vi "QUERY_TELEM_ALL.vi"() -> ()   [LabVIEW 2023, in "Clover_Cell.lvlib"]
uses:
  Clover_Cell.lvlib
panel:
  out "AiP_8":dbl format="%#6.2f"
  out "AiP_7":dbl format="%#6.2f"
  out "AiP_6":dbl format="%#6.2f"
  out "AiP_5":dbl format="%#6.2f"
  out "AiP_4":dbl format="%#6.2f"
  out "AiP_3":dbl format="%#6.2f"
  out "AiP_2":dbl format="%#6.2f"
  out "AiP_1":dbl format="%#2.2f"
  out "Channel_56":i32
  out "Channel_55":i32
  out "Channel_54":i32
  out "Channel_53":i32
  out "Channel_52":i32
  out "Channel_51":i32
  out "Channel_50":i32
  out "Channel_49":i32
  out "Channel_40":i32
  out "Channel_39":i32
  out "Channel_38":i32
  out "Channel_37":i32
  out "Channel_36":i32
  out "Channel_35":i32
  out "Channel_34":i32
  out "Channel_33":i32
  out "Channel_24":i32
  out "Channel_23":i32
  out "Channel_22":i32
  out "Channel_21":i32
  out "Channel_20":i32
  out "Channel_19":i32
  out "Channel_18":i32
  out "Channel_17":i32
  out "Channel_8":i32
  out "Channel_7":i32
  out "Channel_6":i32
  out "Channel_5":i32
  out "Channel_4":i32
  out "Channel_3":i32
  out "Channel_2":i32
  out "Channel_1":i32
  out "L2_Pdet_Array":T1(array[cluster])
  in  "TRXmode":u16(ring)=1 items=["QUERY_TELEM_2 (V)"=2, "QUERY_TELEM_1 (H)"=1]
  in  "TCPIPin":T2={"address"="192.168.100.111", "remote port or service name"=5025, "timeout ms (60000)"=10000}
  out "size(s)":i32
  # "CLC_Gen4_L2"
  # "AiP_1 : 0\nAiP_2 : 1\nAiP_3 : 2\nAiP_4 : 3\nAiP_5 : 4\nAiP_6 : 5\nAiP_7 : 6\nAiP_8 : 7"
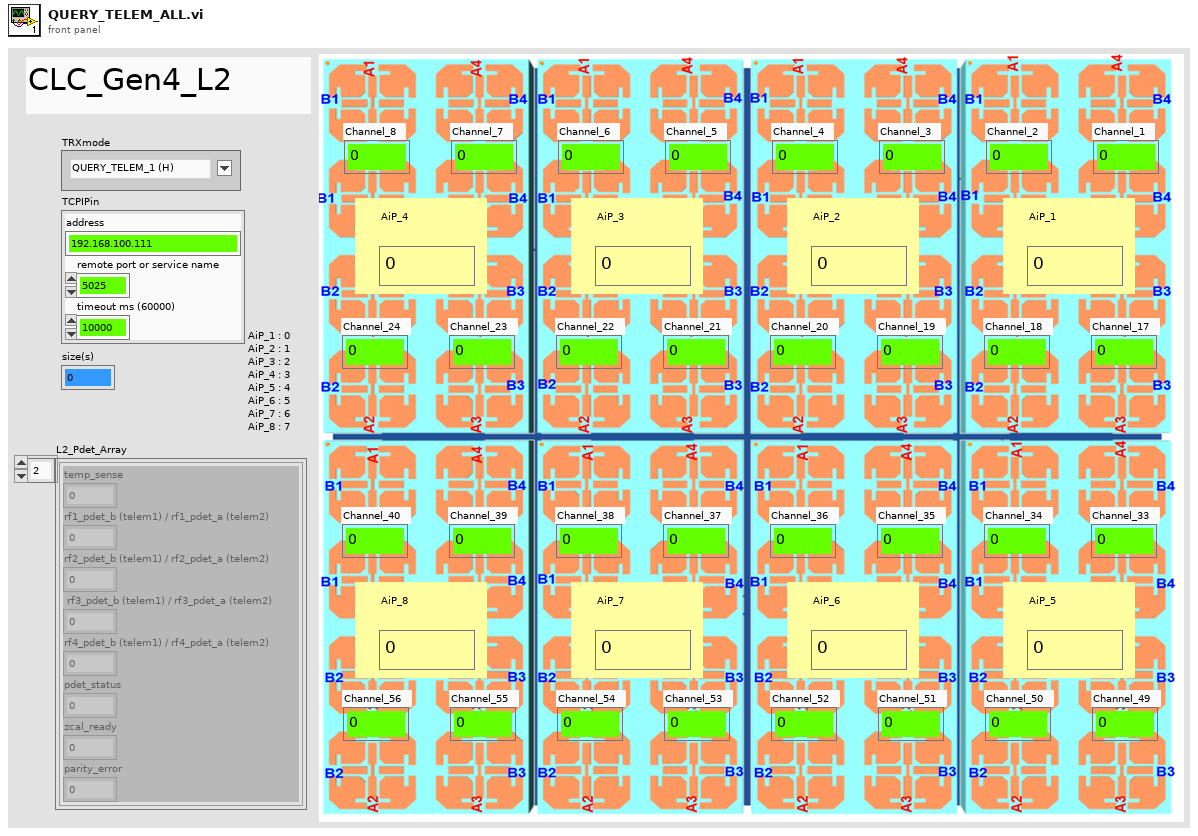
[diagram p1: front panel]
types:
  T1 = cluster{"temp_sense":i32, "rf1_pdet_b (telem1) / rf1_pdet_a (telem2)":i32, "rf2_pdet_b (telem1) / rf2_pdet_a (telem2)":i32, " rf3_pdet_b (telem1) / rf3_pdet_a (telem2)":i32, "rf4_pdet_b (telem1) / rf4_pdet_a (telem2)":i32, "pdet_status":i32, "zcal_ready":i32, "parity_error":i32}[]
  T2 = cluster{"address":string, "remote port or service name":u16, "timeout ms (60000)":i32}
  T3 = cluster{"temp_sense":i32, "rf1_pdet_b (telem1) / rf1_pdet_a (telem2)":i32, "rf2_pdet_b (telem1) / rf2_pdet_a (telem2)":i32, " rf3_pdet_b (telem1) / rf3_pdet_a (telem2)":i32, "rf4_pdet_b (telem1) / rf4_pdet_a (telem2)":i32, "pdet_status":i32, "zcal_ready":i32, "parity_error":i32}
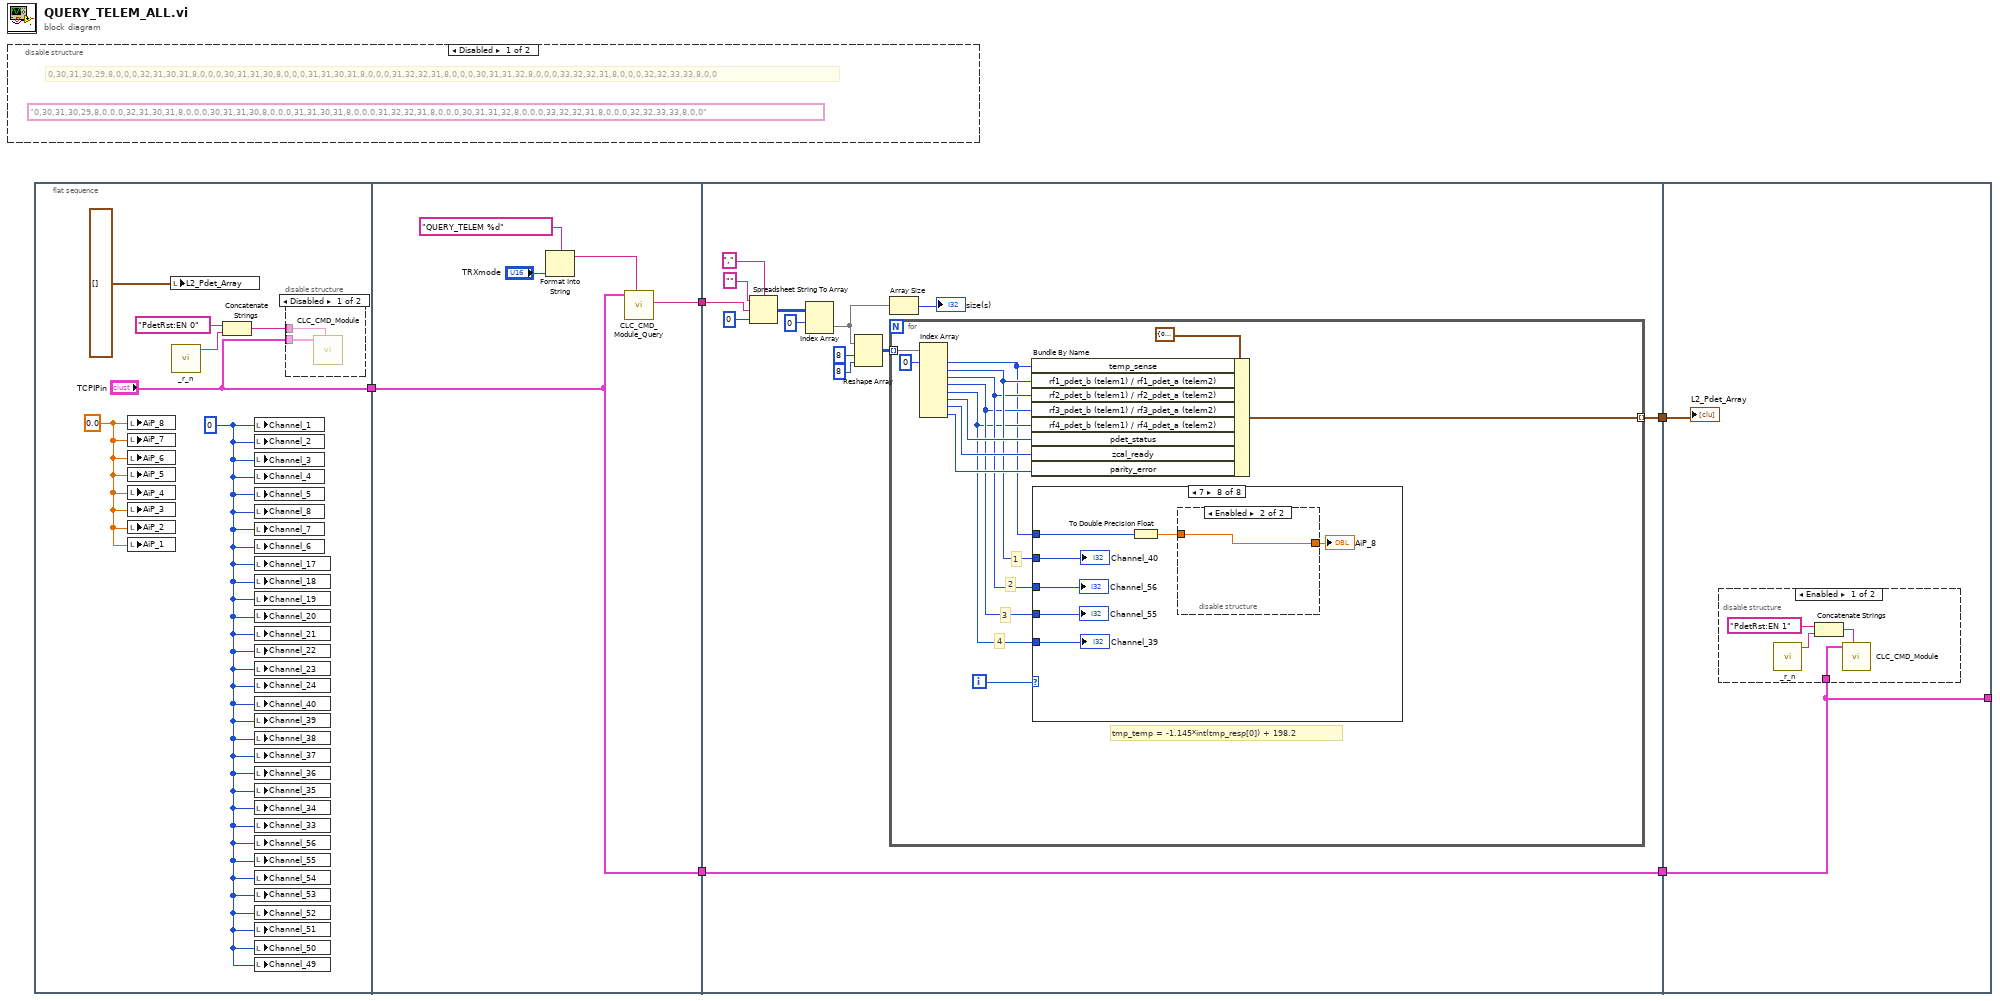
[diagram p0: block diagram]
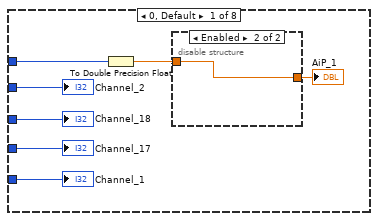
[diagram p4: hidden frame]
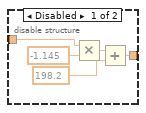
[diagram p5: hidden frame]
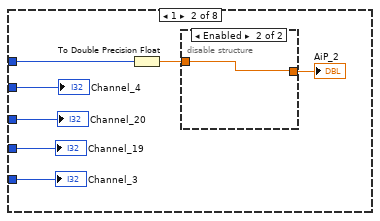
[diagram p6: hidden frame]
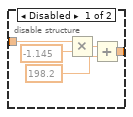
[diagram p7: hidden frame]
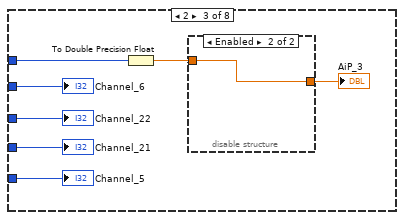
[diagram p8: hidden frame]
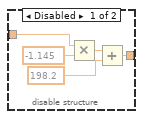
[diagram p9: hidden frame]
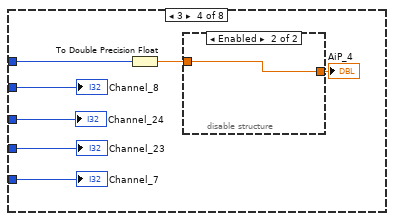
[diagram p10: hidden frame]
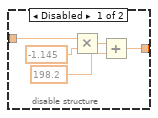
[diagram p11: hidden frame]
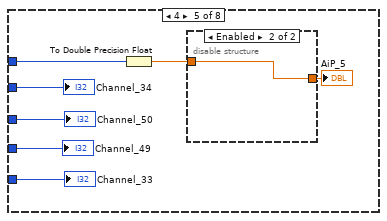
[diagram p12: hidden frame]
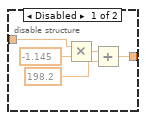
[diagram p13: hidden frame]
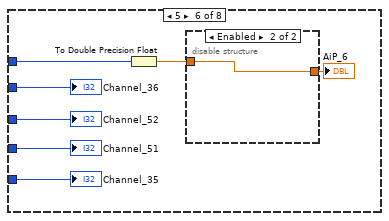
[diagram p14: hidden frame]
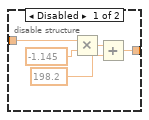
[diagram p15: hidden frame]
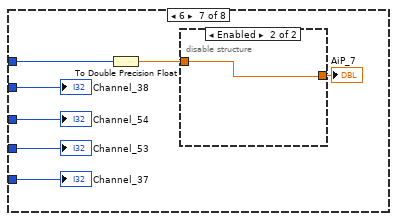
[diagram p16: hidden frame]
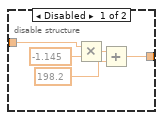
[diagram p17: hidden frame]
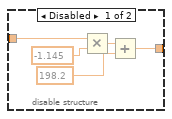
[diagram p18: hidden frame]
diagram:
  n1 = disable-structure shown="Disabled" {
    frame Disabled {
      (unwired) "0,30,31,30,29,8,0,0,0,32,31,30,31,8,0,0,0,30,31,31,30,8,0,0,0,31,31,30,31,8,0,0,0,31,32,32,31,8,0,0,0,30,31,31,32,8,0,0,0,33,32,32,31,8,0,0,0,32,32,33,33,8,0,0"
      # "0,30,31,30,29,8,0,0,0,32,31,30,31,8,0,0,0,30,31,31,30,8,0,0,0,31,31,30,31,8,0,0,0,31,32,32,31,8,0,0,0,30,31,31,32,8,0,0,0,33,32,32,31,8,0,0,0,32,32,33,33,8,0,0"
    }
    frame Enabled {
    }
  }
  n2 = flat-sequence {
    tunnel: ["TCPIPin"] -> w3
    tunnel: [w19] -> w5
    tunnel: [w15] -> w4
    tunnel: w3 -> [w15]
    tunnel: w5 -> [w30]
    tunnel: w4 -> [w21]
    tunnel: [w21] -> w2
    tunnel: [w20] -> w1
    tunnel: [w151] -> _
    tunnel: w2 -> [w151]
    tunnel: w1 -> [w150]
    frame #0 {
      w6 = 0.0 ("AiP_8")
      w7 = 0 ("Channel_1")
      n3 = local write "AiP_8"(w6) -> ()
      n4 = local write "AiP_7"(w6) -> ()
      n5 = local write "AiP_6"(w6) -> ()
      n6 = local write "AiP_5"(w6) -> ()
      n7 = local write "AiP_4"(w6) -> ()
      n8 = local write "AiP_3"(w6) -> ()
      n9 = local write "AiP_2"(w6) -> ()
      n10 = local write "AiP_1"(w6) -> ()
      n11 = local write "L2_Pdet_Array"(T1 [] ("L2")) -> ()
      n12 = call "_r_n.vi"() -> ("command"=w11:string)  [unwired: 5 in]
      n13 = Concatenate Strings("PdetRst:EN 0" ("CMD in"), w11) -> (w10:string)
      n14 = local write "Channel_1"(w7) -> ()
      n15 = local write "Channel_2"(w7) -> ()
      n16 = local write "Channel_3"(w7) -> ()
      n17 = local write "Channel_4"(w7) -> ()
      n18 = local write "Channel_5"(w7) -> ()
      n19 = local write "Channel_8"(w7) -> ()
      n20 = local write "Channel_7"(w7) -> ()
      n21 = local write "Channel_6"(w7) -> ()
      n22 = local write "Channel_17"(w7) -> ()
      n23 = local write "Channel_18"(w7) -> ()
      n24 = local write "Channel_19"(w7) -> ()
      n25 = local write "Channel_20"(w7) -> ()
      n26 = local write "Channel_21"(w7) -> ()
      n27 = local write "Channel_22"(w7) -> ()
      n28 = local write "Channel_23"(w7) -> ()
      n29 = local write "Channel_24"(w7) -> ()
      n30 = local write "Channel_40"(w7) -> ()
      n31 = local write "Channel_39"(w7) -> ()
      n32 = local write "Channel_38"(w7) -> ()
      n33 = local write "Channel_37"(w7) -> ()
      n34 = local write "Channel_36"(w7) -> ()
      n35 = local write "Channel_35"(w7) -> ()
      n36 = local write "Channel_34"(w7) -> ()
      n37 = local write "Channel_33"(w7) -> ()
      n38 = local write "Channel_56"(w7) -> ()
      n39 = local write "Channel_55"(w7) -> ()
      n40 = local write "Channel_54"(w7) -> ()
      n41 = local write "Channel_53"(w7) -> ()
      n42 = local write "Channel_52"(w7) -> ()
      n43 = local write "Channel_51"(w7) -> ()
      n44 = local write "Channel_50"(w7) -> ()
      n45 = local write "Channel_49"(w7) -> ()
      n46 = disable-structure shown="Disabled" {
        disable-tunnel: w10 -> [w14 _]
        disable-tunnel: "TCPIPin" -> [w13 _]
        frame Disabled {
          n47 = call "CLC_CMD_Module.vi"("CMD in"=w14, "TCPIPin"=w13) -> ()  [unwired: 6 in, 4 out]
        }
        frame Enabled {
        }
      }
    }
    frame #1 {
      n48 = Format Into String(format string="QUERY_TELEM %d" ("data in"), "TRXmode") -> (resulting string=w16:string)  [unwired: 2 in, 1 out]
      n49 = call "CLC_CMD_Module_Query.vi"("CMD in"=w16, "TCPIPin"=w15) -> ("data out"=w19:string)  [unwired: 7 in, 2 out]
    }
    frame #2 {
      n50 = Spreadsheet String To Array(delimiter (Tab)=",", format string="", spreadsheet string=w30, array type (2D Dbl)=0) -> (array=w26:i32[][])
      n51 = Index Array(array=w26, index (row)=0 ("disabled index (col)")) -> (element=w24:i32[])  [unwired: 1 in]
      n52 = Reshape Array(w24, 8 ("dimension size"), 8 ("dimension size")) -> (w22:i32[][])
      n53 = Array Size(array=w24) -> (size(s)=→"size(s)":i32)
      n54 = for {
        tunnel: w22 -> [w45] mode=indexing
        tunnel: [w39] -> w20 mode=indexing
        i -> [w38]
        # "tmp_temp = -1.145*int(tmp_resp[0]) + 198.2"
        # "4"
        # "3"
        # "2"
        # "1"
        n55 = Index Array(array=w45, index #1=0 ("index")) -> (element #1=w33:i32, element #2=w37:i32, element #3=w36:i32, element #4=w35:i32, element #5=w34:i32, element #6=w42:i32, element #7=w41:i32, element #8=w40:i32)  [unwired: 7 in]
        n56 = Bundle By Name(cluster=T3 {"temp_sense"=0, "rf1_pdet_b (telem1) / rf1_pdet_a (telem2)"=0, "rf2_pdet_b (telem1) / rf2_pdet_a (telem2)"=0, " rf3_pdet_b (telem1) / rf3_pdet_a (telem2)"=0, "rf4_pdet_b (telem1) / rf4_pdet_a (telem2)"=0, "pdet_status"=0, "zcal_ready"=0, "parity_error"=0} ("L2 Information"), "temp_sense"=w33, "rf1_pdet_b (telem1) / rf1_pdet_a (telem2)"=w37, "rf2_pdet_b (telem1) / rf2_pdet_a (telem2)"=w36, "rf3_pdet_b (telem1) / rf3_pdet_a (telem2)"=w35, "rf4_pdet_b (telem1) / rf4_pdet_a (telem2)"=w34, "pdet_status"=w42, "zcal_ready"=w41, "parity_error"=w40) -> (w39:T3)
        n57 = case shown="7" w38 {
          tunnel: w37 -> [w52 w65 w78 w91 w104 w117 w130 w143]
          tunnel: w36 -> [w51 w64 w77 w90 w103 w116 w129 w142]
          tunnel: w35 -> [w50 w63 w76 w89 w102 w115 w128 w141]
          tunnel: w34 -> [w49 w62 w75 w88 w101 w114 w127 w140]
          tunnel: w33 -> [w47 w60 w73 w86 w99 w112 w125 w138]
          frame 0, Default {
            n58 = To Double Precision Float(number=w47) -> (double precision float=w48:dbl)
            n59 = disable-structure shown="Enabled" {
              disable-tunnel: w48 -> [w54 w58]
              disable-tunnel: [w53 w58] -> w46
              frame Disabled {
                n60 = Multiply(x=w54, y=-1.145) -> (x*y=w56:dbl)
                n61 = Add(x=w56, y=198.2) -> (x+y=w53:dbl)
              }
              frame Enabled {
              }
            }
            "AiP_1" <- w46
            "Channel_2" <- w52
            "Channel_1" <- w49
            "Channel_18" <- w51
            "Channel_17" <- w50
          }
          frame 1 {
            n62 = To Double Precision Float(number=w60) -> (double precision float=w61:dbl)
            n63 = disable-structure shown="Enabled" {
              disable-tunnel: w61 -> [w70 w71]
              disable-tunnel: [w66 w71] -> w59
              frame Disabled {
                n64 = Multiply(x=w70, y=-1.145) -> (x*y=w68:dbl)
                n65 = Add(x=w68, y=198.2) -> (x+y=w66:dbl)
              }
              frame Enabled {
              }
            }
            "AiP_2" <- w59
            "Channel_4" <- w65
            "Channel_20" <- w64
            "Channel_19" <- w63
            "Channel_3" <- w62
          }
          frame 2 {
            n66 = To Double Precision Float(number=w73) -> (double precision float=w74:dbl)
            n67 = disable-structure shown="Enabled" {
              disable-tunnel: w74 -> [w83 w84]
              disable-tunnel: [w79 w84] -> w72
              frame Disabled {
                n68 = Multiply(x=w83, y=-1.145) -> (x*y=w81:dbl)
                n69 = Add(x=w81, y=198.2) -> (x+y=w79:dbl)
              }
              frame Enabled {
              }
            }
            "AiP_3" <- w72
            "Channel_22" <- w77
            "Channel_21" <- w76
            "Channel_6" <- w78
            "Channel_5" <- w75
          }
          frame 3 {
            n70 = To Double Precision Float(number=w86) -> (double precision float=w87:dbl)
            n71 = disable-structure shown="Enabled" {
              disable-tunnel: w87 -> [w96 w97]
              disable-tunnel: [w92 w97] -> w85
              frame Disabled {
                n72 = Multiply(x=w96, y=-1.145) -> (x*y=w94:dbl)
                n73 = Add(x=w94, y=198.2) -> (x+y=w92:dbl)
              }
              frame Enabled {
              }
            }
            "AiP_4" <- w85
            "Channel_8" <- w91
            "Channel_24" <- w90
            "Channel_23" <- w89
            "Channel_7" <- w88
          }
          frame 4 {
            n74 = To Double Precision Float(number=w99) -> (double precision float=w100:dbl)
            n75 = disable-structure shown="Enabled" {
              disable-tunnel: w100 -> [w109 w110]
              disable-tunnel: [w105 w110] -> w98
              frame Disabled {
                n76 = Multiply(x=w109, y=-1.145) -> (x*y=w107:dbl)
                n77 = Add(x=w107, y=198.2) -> (x+y=w105:dbl)
              }
              frame Enabled {
              }
            }
            "AiP_5" <- w98
            "Channel_34" <- w104
            "Channel_50" <- w103
            "Channel_49" <- w102
            "Channel_33" <- w101
          }
          frame 5 {
            n78 = To Double Precision Float(number=w112) -> (double precision float=w113:dbl)
            n79 = disable-structure shown="Enabled" {
              disable-tunnel: w113 -> [w122 w123]
              disable-tunnel: [w118 w123] -> w111
              frame Disabled {
                n80 = Multiply(x=w122, y=-1.145) -> (x*y=w120:dbl)
                n81 = Add(x=w120, y=198.2) -> (x+y=w118:dbl)
              }
              frame Enabled {
              }
            }
            "AiP_6" <- w111
            "Channel_36" <- w117
            "Channel_52" <- w116
            "Channel_51" <- w115
            "Channel_35" <- w114
          }
          frame 6 {
            n82 = To Double Precision Float(number=w125) -> (double precision float=w126:dbl)
            n83 = disable-structure shown="Enabled" {
              disable-tunnel: w126 -> [w135 w136]
              disable-tunnel: [w131 w136] -> w124
              frame Disabled {
                n84 = Multiply(x=w135, y=-1.145) -> (x*y=w133:dbl)
                n85 = Add(x=w133, y=198.2) -> (x+y=w131:dbl)
              }
              frame Enabled {
              }
            }
            "AiP_7" <- w124
            "Channel_38" <- w130
            "Channel_54" <- w129
            "Channel_53" <- w128
            "Channel_37" <- w127
          }
          frame 7 {
            n86 = To Double Precision Float(number=w138) -> (double precision float=w139:dbl)
            n87 = disable-structure shown="Enabled" {
              disable-tunnel: w139 -> [w148 w149]
              disable-tunnel: [w144 w149] -> w137
              frame Disabled {
                n88 = Multiply(x=w148, y=-1.145) -> (x*y=w146:dbl)
                n89 = Add(x=w146, y=198.2) -> (x+y=w144:dbl)
              }
              frame Enabled {
              }
            }
            "AiP_8" <- w137
            "Channel_40" <- w143
            "Channel_56" <- w142
            "Channel_55" <- w141
            "Channel_39" <- w140
          }
        }
      }
    }
    frame #3 {
      n90 = disable-structure shown="Enabled" {
        disable-tunnel: w151 -> [w152 _]
        frame Enabled {
          n91 = call "_r_n.vi"() -> ("command"=w154:string)  [unwired: 5 in]
          n92 = Concatenate Strings("PdetRst:EN 1" ("CMD in"), w154) -> (w155:string)
          n93 = call "CLC_CMD_Module.vi"("CMD in"=w155, "TCPIPin"=w152) -> ()  [unwired: 6 in, 4 out]
        }
        frame Disabled {
        }
      }
      "L2_Pdet_Array" <- w150
    }
  }
